vi "AE Upper Off Angle.vi"(9 "Results 2":T1(array[cluster]) {"Normalized Center"."x" format="%#_2g"; "Normalized Center"."y" format="%#_2g"; "Overall Score" format="%#_2g"; "Distance (ft)" format="%#_3g"; "Area Score" format="%#_2g"; "Moment Score" format="%#_2g"; "Aspect Score" format="%#_2g"}, 11 "Upper Off Angle":dbl) -> (3 "Upper Off Angle Out":dbl)   [LabVIEW 2019]
uses:
  <vilib>/Rock Robotics/Network Tables/NT Write Number.vi
panel:
  # "Scores"
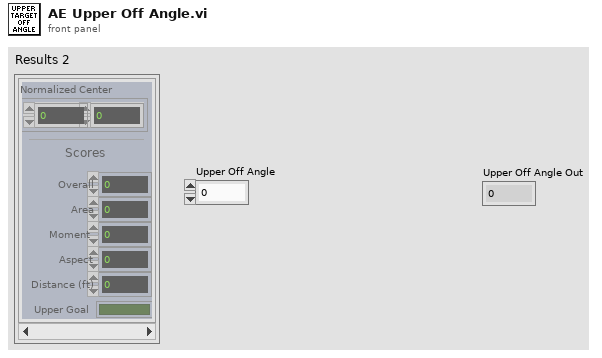
[diagram p1: front panel]
types:
  T1 = cluster{"diameter points":cluster{"first point":cluster{"x":dbl, "y":dbl}, "projected point":cluster{"x":dbl, "y":dbl}}, "Normalized Center":cluster{"x":dbl, "y":dbl}, "Overall Score":dbl, "Area Score":dbl, "Moment Score":dbl, "Aspect Score":dbl, "Distance (ft)":dbl, "Upper Goal":bool}[]
  T2 = cluster{"diameter points":cluster{"first point":cluster{"x":dbl, "y":dbl}, "projected point":cluster{"x":dbl, "y":dbl}}, "Normalized Center":cluster{"x":dbl, "y":dbl}, "Overall Score":dbl, "Area Score":dbl, "Moment Score":dbl, "Aspect Score":dbl, "Distance (ft)":dbl, "Upper Goal":bool}
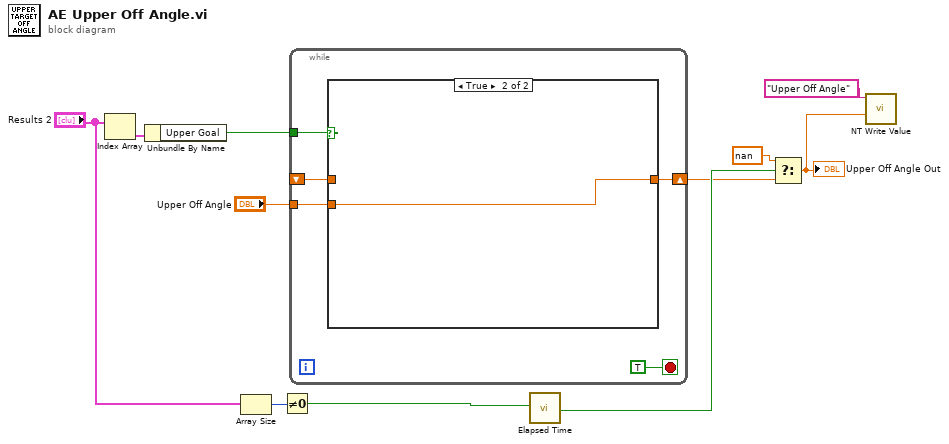
[diagram p0: block diagram]
diagram:
  n1 = Index Array(array="Results 2") -> (element=w10:T2)  [unwired: 1 in]
  n2 = Unbundle By Name(w10) -> ("Upper Goal"=w9:bool)
  n3 = Array Size(array="Results 2") -> (size(s)=w7:i32)
  n4 = Not Equal To 0?(x=w7) -> (x != 0?=w5:bool)
  n5 = while {
    tunnel: w9 -> [w16]
    shift-right: [w15] -> w3
    shift-left: _ -> [w13]
    tunnel: "Upper Off Angle" -> [w14]
    stop <- TRUE stop-if-true
    n6 = case shown="True" w16 {
      tunnel: [w17 w18] -> w15
      tunnel: w14 -> [_ w18]
      tunnel: w13 -> [w17 _]
      frame False {
      }
      frame True {
      }
    }
  }
  n7 = call "Elapsed Time"("Reset"=w5) -> ("Time has Elapsed"=w4:bool)  [unwired: 11 in, 7 out]
  n8 = Select(t=nan, s=w4, f=w3) -> (s? t:f=w1:dbl)
  "Upper Off Angle Out" <- w1
  n9 = call-poly <vilib>:"NT Write Value.vi"("Numeric"=w1, "Name"="Upper Off Angle") -> ()  [unwired: 9 in, 1 out]
